vi "S2C_CMD_FindType.vi"(8 "Error In":errorcluster, 10 "Index":i32, 11 "TypeString":string) -> (0 "Error Out":errorcluster, 1 "AllValues":string[](array[string]), 2 "Value_Int":string, 3 "Value_Text":string, 5 "Found?":bool)   [LabVIEW 2015]
doc: "Returns the Text and Int values for a command Type."
uses:
  S2C_CMD_Globals.vi
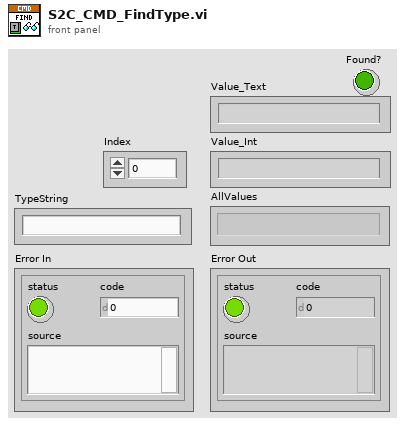
[diagram p1: front panel]
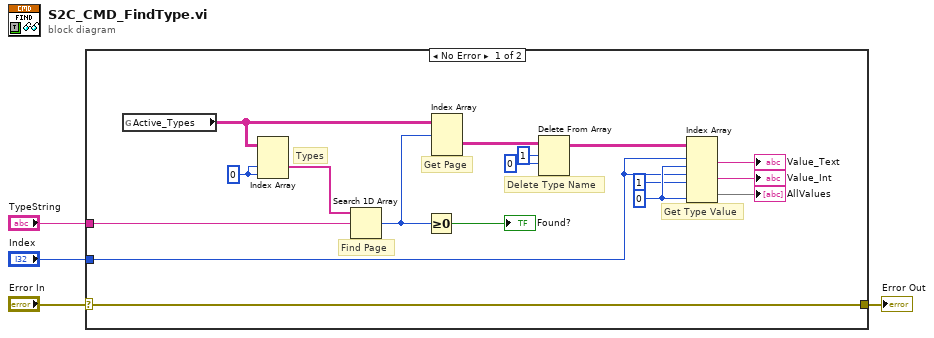
[diagram p0: block diagram]
diagram:
  n1 = case shown="No Error" "Error In" {
    selector: "Error In" -> [w14 w22]
    tunnel: "TypeString" -> [w21 _]
    tunnel: [w14 w22] -> w2
    tunnel: "Index" -> [w7 _]
    frame No Error {
      w9 = 0 ("disabled index (col)")
      w18 = 0 ("disabled index (row)")
      # "Get Type Value"
      # "Delete Type Name"
      # "Get Page"
      # "Find Page"
      # "Types"
      n2 = global read "S2C_CMD_Globals.vi" "Active_Types"() -> (w10:string[][][])
      n3 = Index Array(array=w10, index (dim 1)=w18, index (dim 2)=w18) -> (element=w17:string[])  [unwired: 1 in]
      n4 = Search 1D Array(1D array=w17, element=w21) -> (index of element=w12:i32)  [unwired: 1 in]
      n5 = Greater Or Equal To 0?(x=w12) -> (x >= 0?=→"Found?":bool)
      n6 = Index Array(array=w10, index (dim 0)=w12) -> (element=w16:string[][])  [unwired: 2 in]
      n7 = Delete From Array(array=w16, length=1, index (row)=0) -> (array with subset deleted=w13:string[][])  [unwired: 1 in, 1 out]
      n8 = Index Array(array=w13, index (row) #1=w7, index (col) #1=w9, index (row) #2=w7, index (col) #2=1 ("disabled index (col)"), index (col) #3=w9) -> (element #1=→"Value_Text":string, element #2=→"Value_Int":string, element #3=→"AllValues":string[])  [unwired: 1 in]
    }
    frame Error {
    }
  }
  "Error Out" <- w2
